vi "Power Monitor.vi"(1 "error in":errorcluster) -> (0 "error out":errorcluster)   [LabVIEW 2017]
uses:
  <vilib>/Rock Robotics/Network Tables/NT Write Numeric Array.vi
  <vilib>/Rock Robotics/Network Tables/NT Write Number.vi
panel:
  out "Solenoid Voltage":dbl
  out "PCM Input Voltage":dbl
  out "Compress Current (Amps)":dbl
  out "Max Wheel Current":i32
  out "Wheel Current (Amps)":dbl
  out "calculated Amp":dbl
  out "Total Amps of All Channels":dbl
  out "PDP Total Current":dbl[](array[numeric])
  out "Power (W)":dbl
  out "voltage (V)":dbl
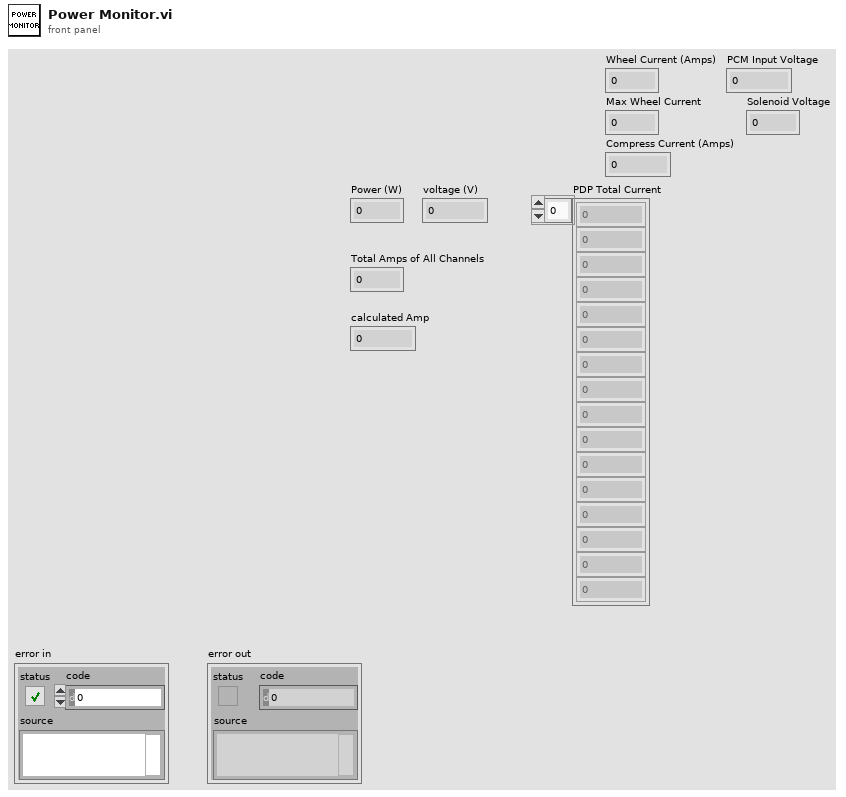
[diagram p1: front panel]
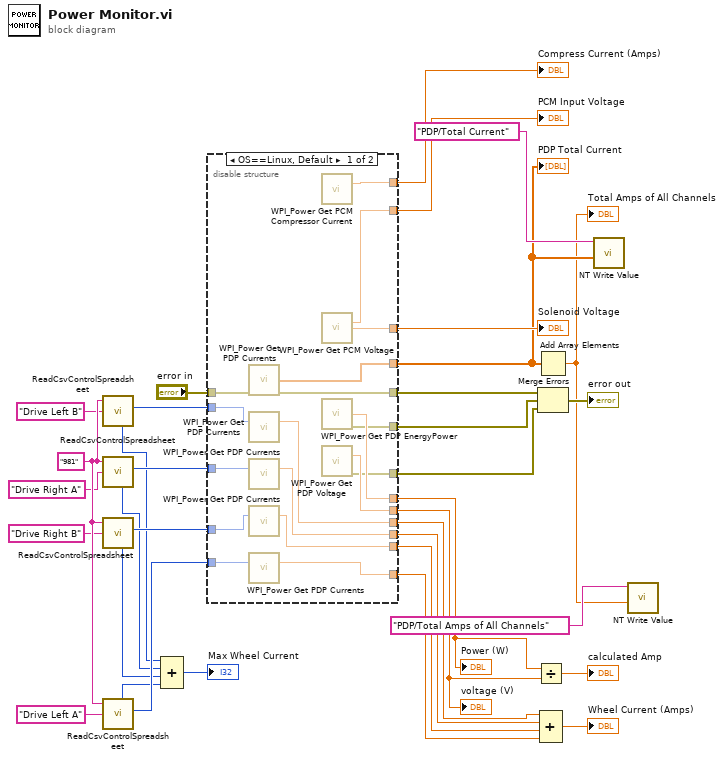
[diagram p0: block diagram]
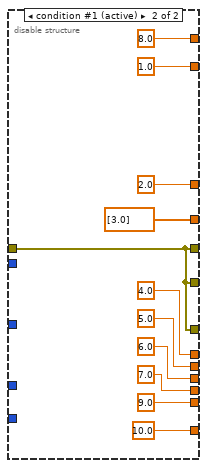
[diagram p2: hidden frame]
diagram:
  w29 = "981" ("Robot ID")
  n1 = call "ReadCsvControlSpreadsheet.vi"("Robot ID"=w29, "Motor ID"="Drive Left B") -> ("PDP Channel ID"=w24:i32, "Max Allowed Current"=w15:i32)  [unwired: 1 in, 3 out]
  n2 = call "ReadCsvControlSpreadsheet.vi"("Robot ID"=w29, "Motor ID"="Drive Right A") -> ("PDP Channel ID"=w23:i32, "Max Allowed Current"=w14:i32)  [unwired: 1 in, 3 out]
  n3 = call "ReadCsvControlSpreadsheet.vi"("Robot ID"=w29, "Motor ID"="Drive Right B") -> ("PDP Channel ID"=w22:i32, "Max Allowed Current"=w13:i32)  [unwired: 1 in, 3 out]
  n4 = call "ReadCsvControlSpreadsheet.vi"("Robot ID"=w29, "Motor ID"="Drive Left A") -> ("PDP Channel ID"=w21:i32, "Max Allowed Current"=w12:i32)  [unwired: 1 in, 3 out]
  n5 = Compound Arithmetic op=ADD(w15, w14, w13, w12) -> (→"Max Wheel Current":i32)
  n6 = disable-structure shown="OS==Linux, Default" {
    disable-tunnel: "error in" -> [w52 w63]
    disable-tunnel: [w51 4.0 ("Power (W)")] -> w32
    disable-tunnel: [w50 5.0 ("voltage (V)")] -> w31
    disable-tunnel: w24 -> [w49 _]
    disable-tunnel: w23 -> [w48 _]
    disable-tunnel: w22 -> [w47 _]
    disable-tunnel: w21 -> [w46 _]
    disable-tunnel: [w45 6.0 ("current (A)")] -> w20
    disable-tunnel: [w44 7.0 ("current (A)")] -> w19
    disable-tunnel: [w43 9.0 ("current (A)")] -> w18
    disable-tunnel: [w42 10.0 ("current (A)")] -> w17
    disable-tunnel: [w41 w63] -> w10
    disable-tunnel: [w40 w63] -> w9
    disable-tunnel: [w39 w63] -> w8
    disable-tunnel: [w38 8.0 ("Compress Current (Amps)")] -> w7
    disable-tunnel: [w37 1.0 ("PCM Input Voltage")] -> w6
    disable-tunnel: [w36 2.0 ("Solenoid Voltage")] -> w5
    disable-tunnel: [w35 dbl[] [3.0] ("PDP Total Current")] -> w3
    frame condition #0 {
      n7 = call <vilib>:"WPI_Power Get PDP Currents.vi"("error in"=w52) -> ("all currents (A)"=w35:dbl[], "error out"=w41:errorcluster)  [unwired: 12 in, 1 out]
      n8 = call <vilib>:"WPI_Power Get PDP Currents.vi"("PDP Channel"=w49) -> ("current (A)"=w45:dbl)  [unwired: 12 in, 2 out]
      n9 = call <vilib>:"WPI_Power Get PDP Currents.vi"("PDP Channel"=w48) -> ("current (A)"=w44:dbl)  [unwired: 12 in, 2 out]
      n10 = call <vilib>:"WPI_Power Get PDP Currents.vi"("PDP Channel"=w47) -> ("current (A)"=w43:dbl)  [unwired: 12 in, 2 out]
      n11 = call <vilib>:"WPI_Power Get PDP Currents.vi"("PDP Channel"=w46) -> ("current (A)"=w42:dbl)  [unwired: 12 in, 2 out]
      n12 = call <vilib>:"WPI_Power Get PCM Compressor Current.vi"() -> ("current (A)"=w38:dbl)  [unwired: 14 in, 1 out]
      n13 = call <vilib>:"WPI_Power Get PCM Voltage.vi"() -> ("Input Voltage"=w37:dbl, "Solenoid Voltage"=w36:dbl)  [unwired: 13 in, 1 out]
      n14 = call <vilib>:"WPI_Power Get PDP EnergyPower.vi"() -> ("Power (W)"=w51:dbl, "error out"=w40:errorcluster)  [unwired: 13 in, 1 out]
      n15 = call <vilib>:"WPI_Power Get PDP Voltage.vi"() -> ("voltage (V)"=w50:dbl, "error out"=w39:errorcluster)  [unwired: 14 in]
    }
    frame condition #1 (active) {
    }
  }
  "voltage (V)" <- w31
  "Power (W)" <- w32
  "PDP Total Current" <- w3
  "Compress Current (Amps)" <- w7
  "PCM Input Voltage" <- w6
  "Solenoid Voltage" <- w5
  n16 = Divide(x=w32, y=w31) -> (x/y=→"calculated Amp":dbl)
  n17 = Add Array Elements(numeric array=w3) -> (sum=w1:dbl)
  "Total Amps of All Channels" <- w1
  n18 = Merge Errors(w10, w9, w8) -> (→"error out":errorcluster)
  n19 = Compound Arithmetic op=ADD(w20, w19, w18, w17) -> (→"Wheel Current (Amps)":dbl)
  n20 = call-poly <vilib>:"NT Write Value.vi"("Numeric Array"=w3, "Name"="PDP/Total Current") -> ()  [unwired: 9 in, 1 out]
  n21 = call-poly <vilib>:"NT Write Value.vi"("Numeric"=w1, "Name"="PDP/Total Amps of All Channels") -> ()  [unwired: 9 in, 1 out]
